vi "Init.vi"(8 "error in (no error)":errorcluster, 10 "Index":i32) -> (0 "error out":errorcluster, 3 "Step In Query out":refnum<class "Set Index Query.lvclass">)   [LabVIEW 2013, in "Set Index Query.lvclass"]
doc: "Copyright 2018, Carya Automatisering, Wiebe Walstra."
uses:
  Set Index Query.lvclass
  Set Index Query.lvclass/Set Index Query.ctl
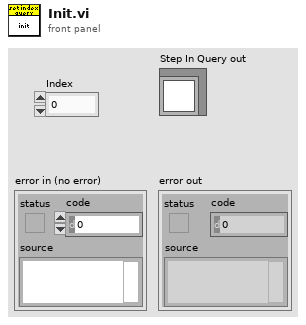
[diagram p1: front panel]
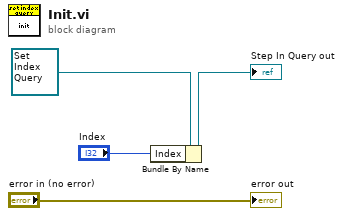
[diagram p0: block diagram]
diagram:
  n1 = Bundle By Name(cluster=refnum<class "Set Index Query.lvclass"> refnum ("Step In Query in"), "Index"="Index") -> (→"Step In Query out":refnum<class "Set Index Query.lvclass">)
  "error out" <- "error in (no error)"
